vi "is cancelled.vi"(11 "cancel token in":refnum<class "cancel token.lvclass">) -> (2 "cancelled?":bool, 3 "cancel token out":refnum<class "cancel token.lvclass">)   [LabVIEW 2013, in "cancel token.lvclass"]
uses:
  cancel token.lvclass
  cancel token.lvclass/cancel token.ctl
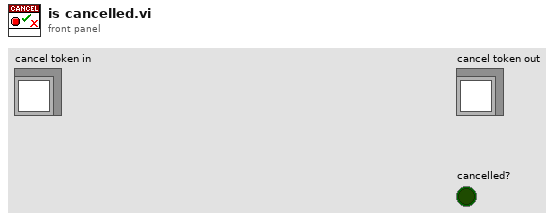
[diagram p1: front panel]
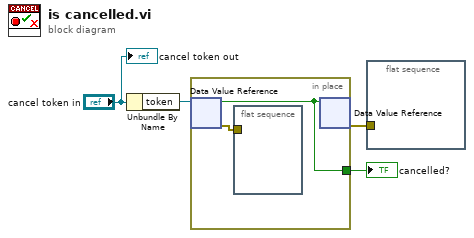
[diagram p0: block diagram]
diagram:
  n1 = Unbundle By Name("cancel token in") -> ("token"=w3:refnum<data-value>)
  n2 = in-place {
    in-place-border: [w6] -> w2
    n3 = in-place-dvr #1(w3) -> (w6:bool, w5:errorcluster)
    n4 = flat-sequence {
      tunnel: w5 -> [_]
      frame #0 {
      }
    }
    n5 = in-place-dvr #1(w6) -> (w1:errorcluster)  [unwired: 1 out]
  }
  "cancelled?" <- w2
  n6 = flat-sequence {
    tunnel: w1 -> [_]
    frame #0 {
    }
  }
  "cancel token out" <- "cancel token in"
